vi "sort.vi"(10 "mius_flash_order":i32[][](array[numeric]), 11 "HRV_data":dbl[](array[numeric])) -> (3 "appended array":dbl[][](array[numeric]))   [LabVIEW 2014]
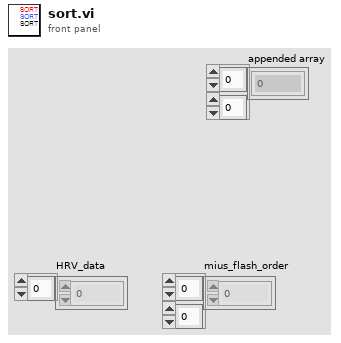
[diagram p1: front panel]
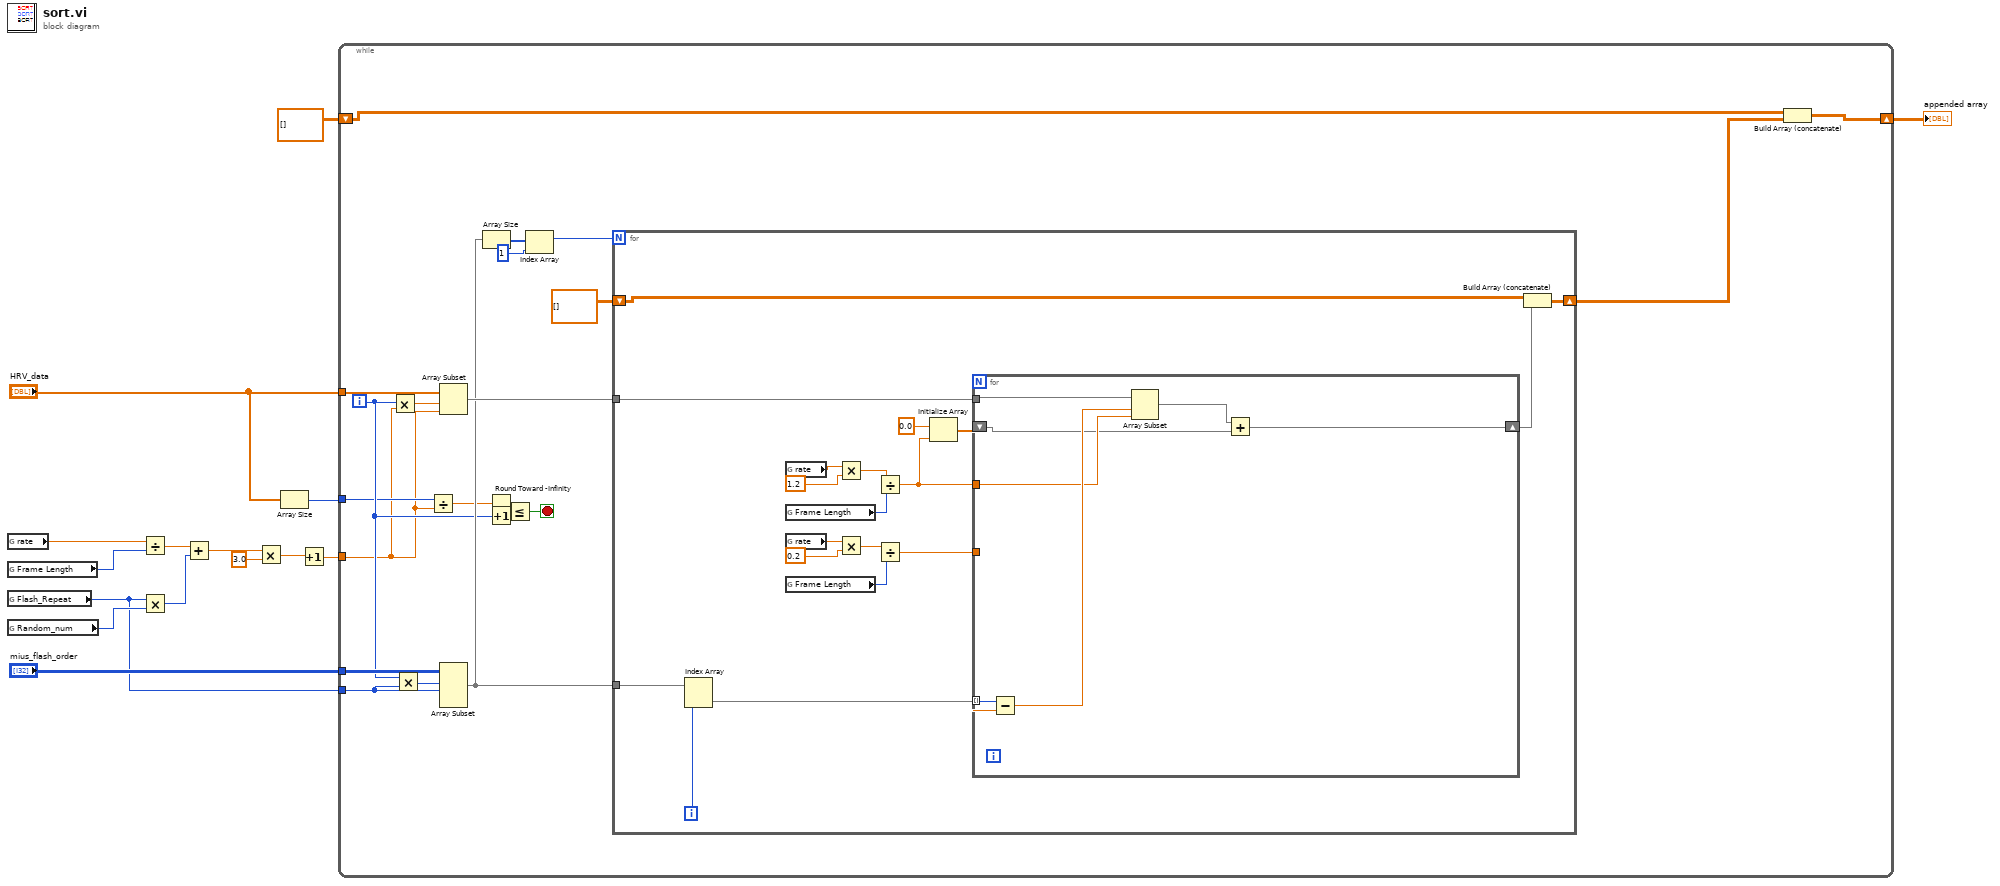
[diagram p0: block diagram]
diagram:
  n1 = global read "Control_Panel.vi" "rate"() -> (w15:dbl)
  n2 = global read "Control_Panel.vi" "Frame Length"() -> (w9:i32)
  n3 = global read "Control_Panel.vi" "Flash_Repeat"() -> (w5:i32)
  n4 = global read "Control_Panel.vi" "Random_num"() -> (w13:i32)
  n5 = Divide(x=w15, y=w9) -> (x/y=w14:dbl)
  n6 = Multiply(x=w5, y=w13) -> (x*y=w12:i32)
  n7 = Add(x=w14, y=w12) -> (x+y=w10:dbl)
  n8 = Multiply(x=w10, y=3.0) -> (x*y=w8:dbl)
  n9 = Array Size(array="HRV_data") -> (size(s)=w4:i32)
  n10 = Increment(x=w8) -> (x+1=w7:dbl)
  n11 = while {
    tunnel: "HRV_data" -> [w36]
    tunnel: w7 -> [w22]
    tunnel: "mius_flash_order" -> [w34]
    tunnel: w5 -> [w32]
    tunnel: w4 -> [w23]
    shift-right: [w17] -> w3
    shift-left: dbl[][] [] -> [w16]
    i -> [w25]
    stop <- w26 stop-if-true
    n12 = Multiply(x=w25, y=w22) -> (x*y=w35:dbl)
    n13 = Multiply(x=w25, y=w32) -> (x*y=w33:i32)
    n14 = Divide(x=w23, y=w22) -> (x/y=w21:dbl)
    n15 = Array Subset(array=w36, index=w35, length=w22) -> (w31:dbl[])
    n16 = Array Subset(array=w34, index (row)=w33, length (row)=w32) -> (w30:i32[][])  [unwired: 2 in]
    n17 = Array Size(array=w30) -> (size(s)=w28:i32[])
    n18 = Round Toward -Infinity(1:w21) -> (0:w20:dbl)
    n19 = Increment(x=w25) -> (x+1=w24:i32)
    n20 = Less Or Equal?(x=w20, y=w24) -> (x <= y?=w26:bool)
    n21 = Index Array(array=w28, index=1 ("인덱스")) -> (element=w27:i32)
    n22 = for {
      N: w27 -> [_]
      tunnel: w31 -> [w53]
      tunnel: w30 -> [w55]
      shift-right: [w38] -> w18
      shift-left: dbl[][] [] -> [w37]
      i -> [w54]
      n23 = Index Array(array=w55, index (col)=w54) -> (element=w52:i32[])  [unwired: 1 in]
      n24 = global read "Control_Panel.vi" "rate"() -> (w46:dbl)
      n25 = global read "Control_Panel.vi" "Frame Length"() -> (w43:i32)
      n26 = global read "Control_Panel.vi" "rate"() -> (w51:dbl)
      n27 = global read "Control_Panel.vi" "Frame Length"() -> (w48:i32)
      n28 = Multiply(x=w46, y=1.2) -> (x*y=w44:dbl)
      n29 = Multiply(x=w51, y=0.2) -> (x*y=w49:dbl)
      n30 = Divide(x=w44, y=w43) -> (x/y=w40:dbl)
      n31 = Divide(x=w49, y=w48) -> (x/y=w47:dbl)
      n32 = Initialize Array(0.0 ("element"), w40) -> (w41:dbl[])
      n33 = for {
        tunnel: w53 -> [w63]
        tunnel: w52 -> [w62] mode=indexing
        tunnel: w47 -> [w61]
        tunnel: w40 -> [w59]
        shift-right: [w57] -> w39
        shift-left: w41 -> [w56]
        n34 = Subtract(x=w62, y=w61) -> (x-y=w60:dbl)
        n35 = Array Subset(array=w63, index=w60, length=w59) -> (w58:dbl[])
        n36 = Add(x=w58, y=w56) -> (x+y=w57:dbl[])
      }
      n37 = Build Array (concatenate)(w37, w39) -> (w38:dbl[][])
    }
    n38 = Build Array (concatenate)(w16, w18) -> (w17:dbl[][])
  }
  "appended array" <- w3
